vi "Min and Max Data.vi"(8 "error in (no error)":errorcluster, 10 "Input (0:A)":u16(ring) items=["A", "B", "C", "D"], 11 "VISA resource name":refnum<visa-resource-name>) -> (0 "error out":errorcluster, 1 "Min Sensor Data":dbl format="%.4f", 2 "Max Sensor Data":dbl format="%.4f", 3 "VISA resource name out":refnum<visa-resource-name>)   [LabVIEW 2021, in "Lake Shore 336.lvlib"]
doc: "This VI returns the status of the Min and Max data for the selected sensor input. The Max/Min feature captures and stores the highest (Max) and lowest (Min) reading taken since the last reset. The Preferred Units parameter, under the Input Setup menu, determines the units used for capturing Max and Min. Max and Min are always being captured, so there is no need to turn the feature on or off. The readings are reset when the instrument is turned off, sendos input parameters are changed, the Max/Min Reset key is pressed, or the Reset Min and Max VI is executed."
uses:
  <instrlib>/Lake Shore 336/Lake Shore 336.lvlib
  Instance           1 24Saved   Min and Max Data .vi
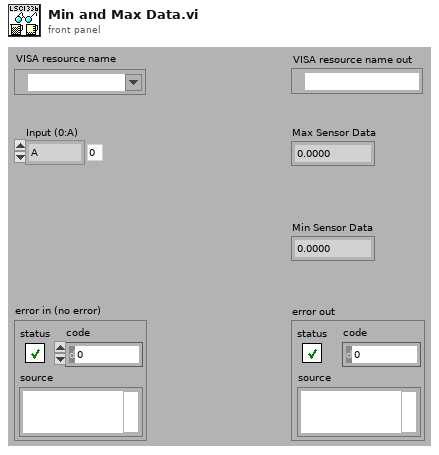
[diagram p1: front panel]
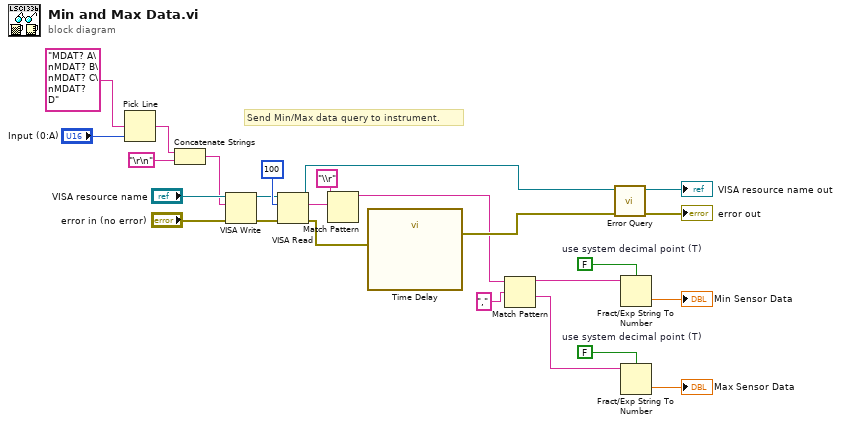
[diagram p0: block diagram]
diagram:
  w4 = FALSE  # use system decimal point (T)
  w6 = FALSE  # use system decimal point (T)
  # "Send Min/Max data query to instrument."
  n1 = Pick Line(multi-line string="MDAT? A\nMDAT? B\nMDAT? C\nMDAT? D", line index="Input (0:A)") -> (output string=w10:string)  [unwired: 1 in]
  n2 = Concatenate Strings(w10, "\r\n") -> (w8:string)
  n3 = VISA Write(VISA resource name="VISA resource name", write buffer=w8, error in (no error)="error in (no error)") -> (VISA resource name out=w14:refnum<visa-resource-name>, error out=w13:errorcluster)  [unwired: 1 out]
  n4 = VISA Read(VISA resource name=w14, byte count=100, error in (no error)=w13) -> (VISA resource name out=w24:refnum<visa-resource-name>, read buffer=w16:string, error out=w12:errorcluster)  [unwired: 1 out]
  n5 = Match Pattern(string=w16, regular expression="\\r") -> (before substring=w7:string)  [unwired: 1 in, 3 out]
  n6 = call "Time Delay"("error in (no error)"=w12) -> ("error out"=w23:errorcluster)  [unwired: 10 in]
  n7 = Match Pattern(string=w7, regular expression=",") -> (before substring=w5:string, after substring=w3:string)  [unwired: 1 in, 2 out]
  n8 = call <instrlib>:"Error Query.vi"("error in (no error)"=w23, "VISA resource name"=w24) -> ("error out"=→"error out":errorcluster, "VISA resource name out"=→"VISA resource name out":refnum<visa-resource-name>)  [unwired: 7 in, 1 out]
  n9 = Fract/Exp String To Number(use system decimal point (T)=w6, string=w5) -> (number=→"Min Sensor Data":dbl)  [unwired: 2 in, 1 out]
  n10 = Fract/Exp String To Number(use system decimal point (T)=w4, string=w3) -> (number=→"Max Sensor Data":dbl)  [unwired: 2 in, 1 out]
